vi "upload.abort_multipart_upload.vi"(8 "error in":errorcluster, 11 "Multipart Upload":refnum<class "Multipart Upload.lvclass">) -> (0 "error out":errorcluster)   [LabVIEW 2020, in "Multipart Upload.lvclass"]
doc: "Aborts a multipart upload to S3. Frees storage used by previously uploaded parts and prevents further uploads to the same uploadId."
uses:
  Multipart Upload.lvclass
  Multipart Upload.lvclass/Multipart Upload.ctl
  nominal_client.get.vi
  Nominal Client/Nominal Client.lvclass
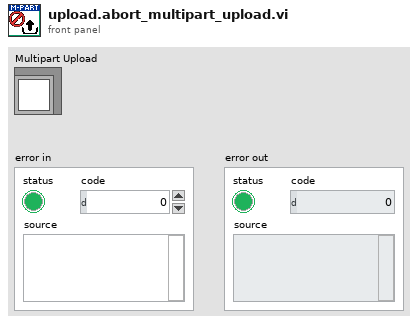
[diagram p1: front panel]
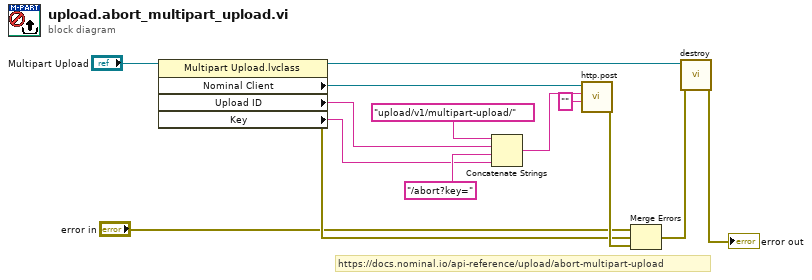
[diagram p0: block diagram]
diagram:
  # "https://docs.nominal.io/api-reference/upload/abort-multipart-upload"
  n1 = property class="Multipart Upload.lvclass"(reference="Multipart Upload") -> (reference out=w4:refnum<class "Multipart Upload.lvclass">, error out=w6:errorcluster, "Nominal Client"=w5:refnum<class "Nominal Client.lvclass">, "Upload ID"=w8:string, "Key"=w7:string)  [unwired: 1 in]
  n2 = Concatenate Strings("upload/v1/multipart-upload/" ("Path"), w8, "/abort?key=" ("string"), w7) -> (w13:string)
  n3 = call "http.post.vi"("Request body"="", "Path"=w13, "Nominal Client in"=w5) -> ("error out"=w10:errorcluster)  [unwired: 6 in, 2 out]
  n4 = Merge Errors("error in", w6, w10) -> (w3:errorcluster)
  n5 = call "destroy.vi"("error in"=w3, "MultiPart Upload"=w4) -> ("error out"=→"error out":errorcluster)  [unwired: 9 in]
